vi "Main.vi"(11 "Module Admin":refnum<class "Delacor_lib_QMH_Module Admin.lvclass">) -> ()   [LabVIEW 2021, in "RT Interpreter.lvlib"]
doc: "This template is based off of the Queued Message Handler design pattern and the Queued Message Handler project template that ships with LabVIEW.\n\nThe main difference is that the queue is private to this module and communication between modules is performed via Broadcast and Request events.\n\nRequest events are wrapped in public API methods and are handled in the Event Handling Loop (EHL) of this VI. Any module can register for Broadcast events sent by this module. The EHL generates messages based on user interface actions.\n\nThe Message Handling Loop (MHL) processes messages generated by the EHL, or by other messages. The messages are string values, so new messages can be added easily to the Message Cases case structure in the MHL. Each message cluster can also provide an optional value for Message Data, which is a variant that can be converted to whatever message-specific data is required.\n_____\nBased on DQMH Dev Tools: Project Template 7.1.2.1547."
uses:
  RT Interpreter.lvlib
  <vilib>/Delacor/Delacor QMH/Libraries/Module Admin_class/Delacor_lib_QMH_Module Admin.lvclass
  Host/Host Interpreter/Host Initialization--cluster.ctl
  Module Data--cluster.ctl
  Stop Argument--cluster.ctl
  <vilib>/Delacor/Delacor QMH/Libraries/Message Queue_class/Delacor_lib_QMH_Message Queue.lvclass/Delacor_lib_QMH_Message Queue.ctl
  <vilib>/Delacor/Delacor QMH/Libraries/Module Admin_class/Delacor_lib_QMH_Module Admin.lvclass/Delacor_lib_QMH_Module Admin.ctl
  189c6fa9-2a90-4507-a0f2-9e31c6cf4c77.vi
  <vilib>/Delacor/Delacor QMH/Libraries/Message Queue_class/Delacor_lib_QMH_Enqueue Message (Single).vi
  <vilib>/Delacor/Delacor QMH/Libraries/Module Admin_class/Delacor_lib_QMH_Get External Launch.vi
  <vilib>/JDP Science/JSONtext/JSON text to Variant.vi
  <vilib>/JDP Science/JSONtext/LVClass Serializer/JSONtext LVClass Serializer.lvclass
  <vilib>/Delacor/Delacor QMH/Libraries/Message Queue_class/Delacor_lib_QMH_Message Queue.lvclass
  Libraries/UDP Comms/UDP Comms.lvlib
panel:
  out "Data out":T1
  out "error out":errorcluster
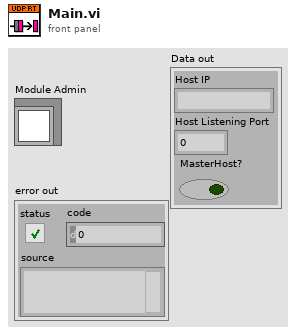
[diagram p1: front panel]
types:
  T1 = typedef "UDP Comms.lvlib/Host Initialization--cluster.ctl" = cluster{"Host IP":string, "Host Listening Port":u16, "MasterHost?":bool}
  T2 = typedef "RT Interpreter.lvlib/Request Events--cluster.ctl" = cluster{"Stop Module":refnum<user-event>, "Show Panel":refnum<user-event>, "Hide Panel":refnum<user-event>, "Get Module Execution Status":refnum<user-event>, "Show Diagram":refnum<user-event>, "Private.Open Connection":refnum<user-event>, "Private.Start Helper Loop":refnum<user-event>}
  T3 = typedef "RT Interpreter.lvlib/Module Data--cluster.ctl" = cluster{"IP Host":string, "Port RT":u16, "Port Host":u16, "connection ID":refnum<k16>}
  T4 = enum32{"invalid lock state", "Not Locked", "Locked (No Password)", "Password-protected"}
  T5 = typedef "RT Interpreter.lvlib/Stop Argument--cluster.ctl" = cluster{"Origin":string, "Exit via Stop Module Req?":bool, "Wait for Module to stop?":bool}
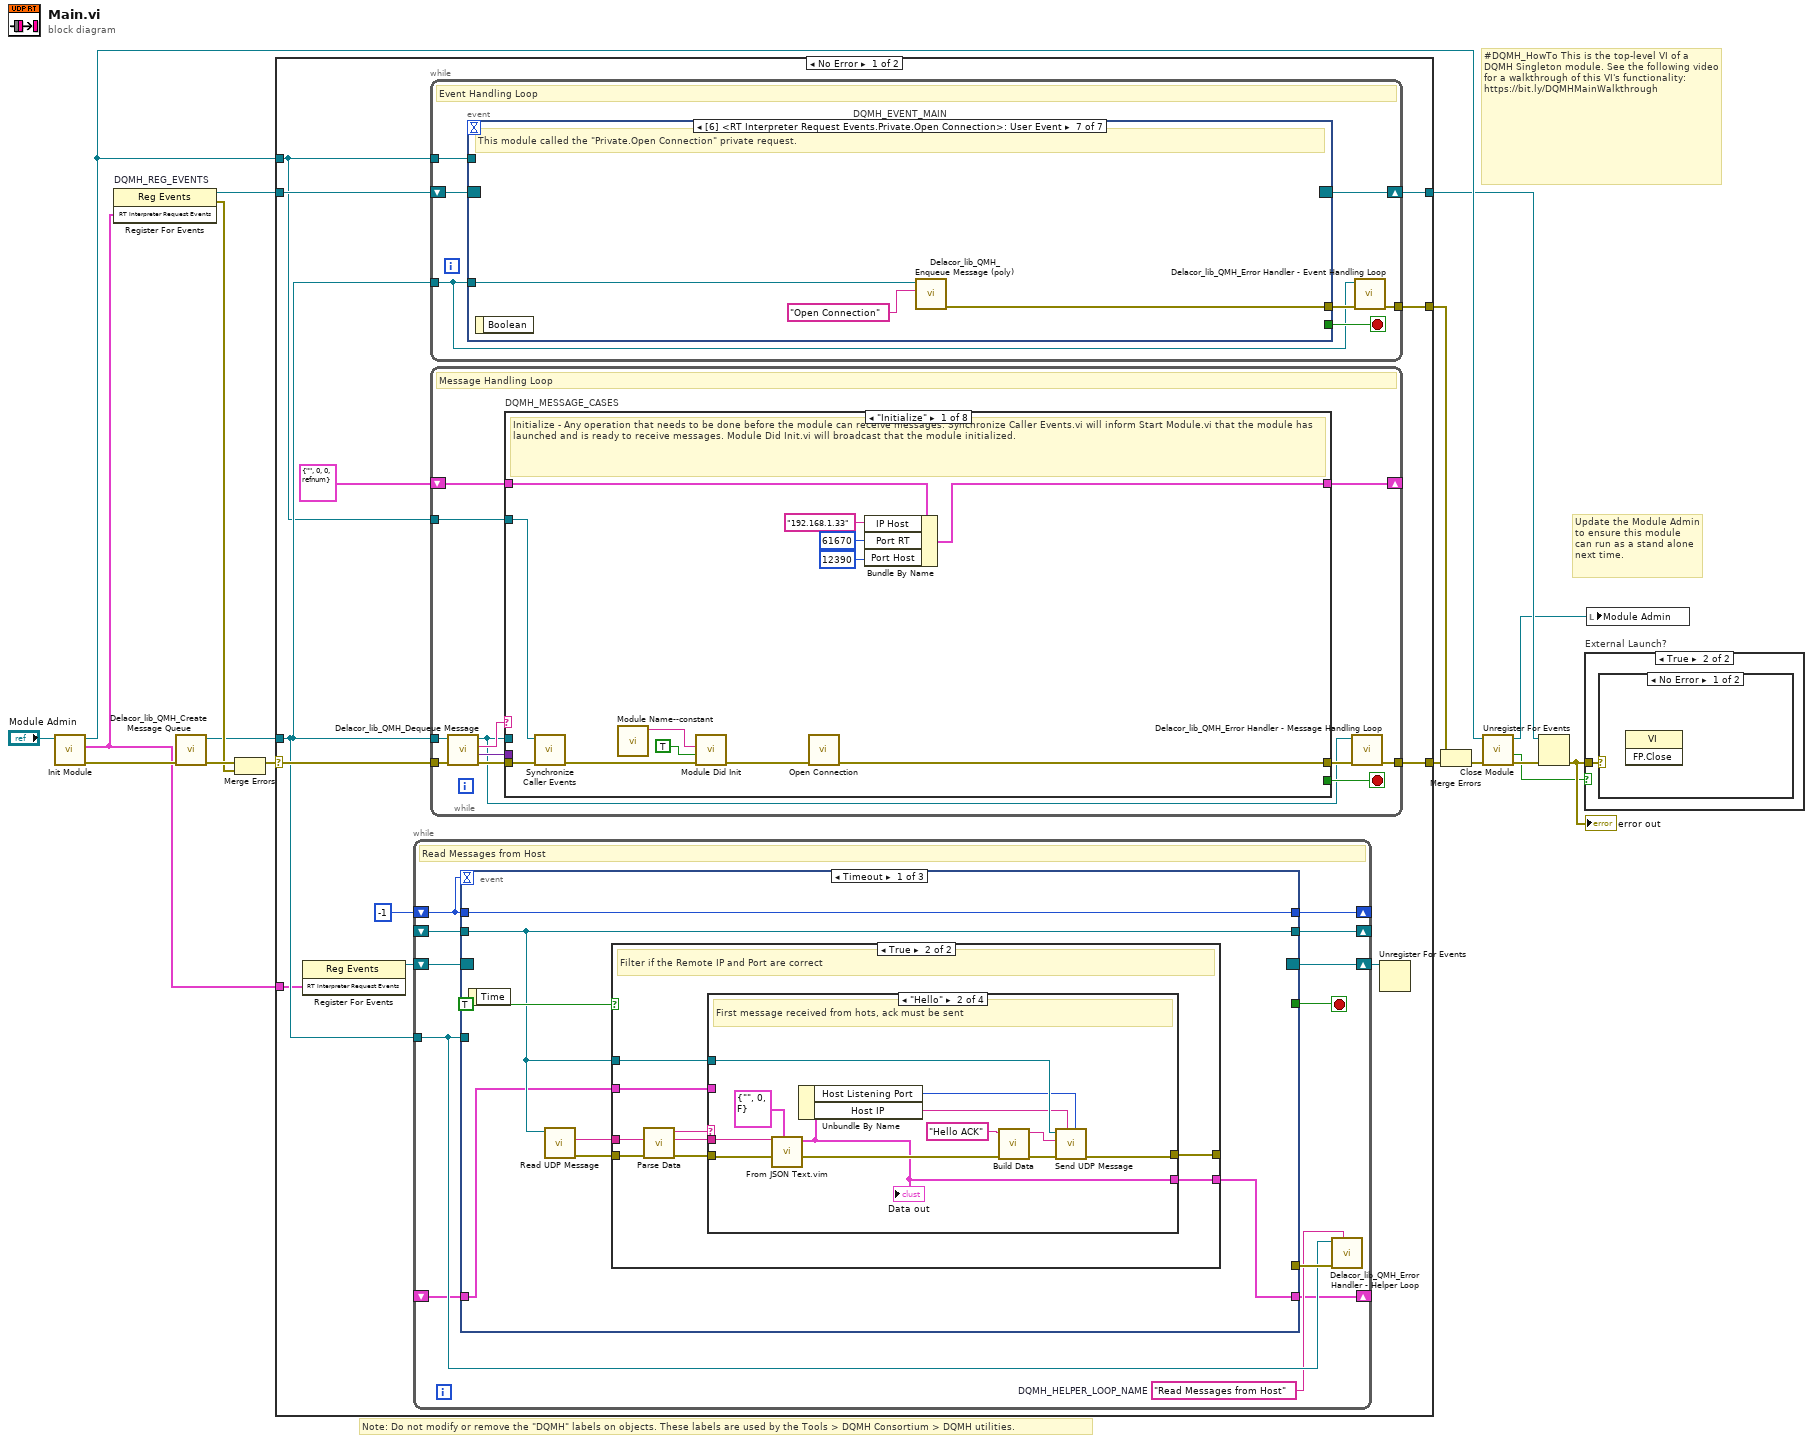
[diagram p0: block diagram]
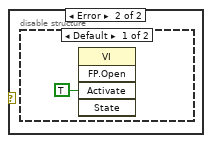
[diagram p3: hidden frame]
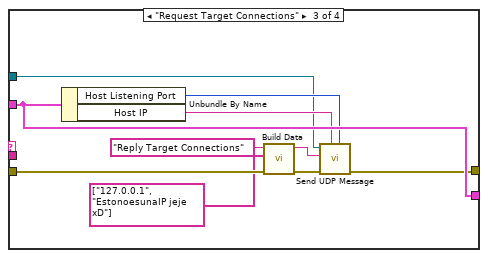
[diagram p7: hidden frame]
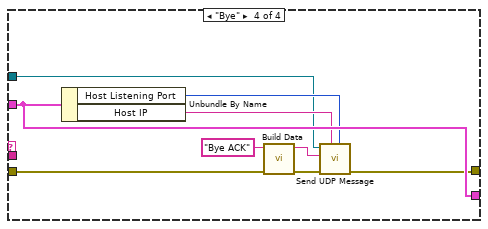
[diagram p8: hidden frame]
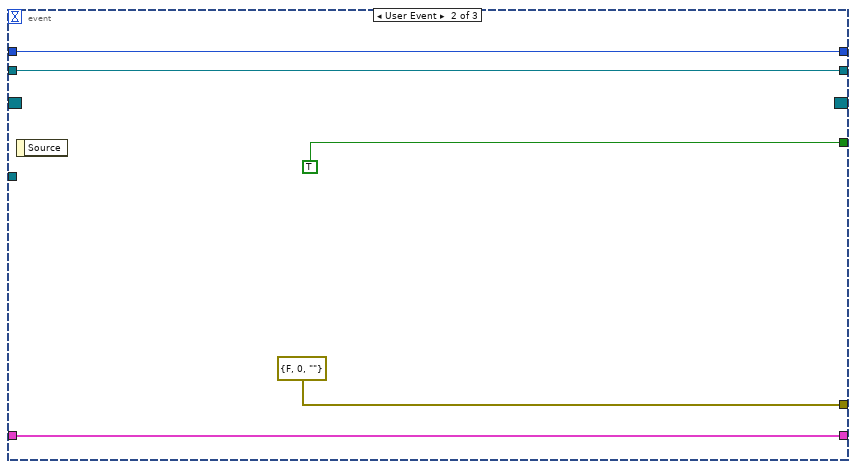
[diagram p9: hidden frame]
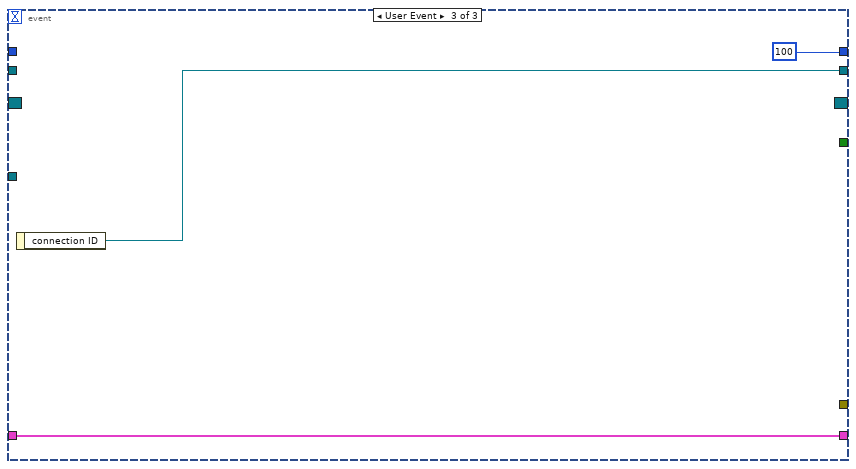
[diagram p10: hidden frame]
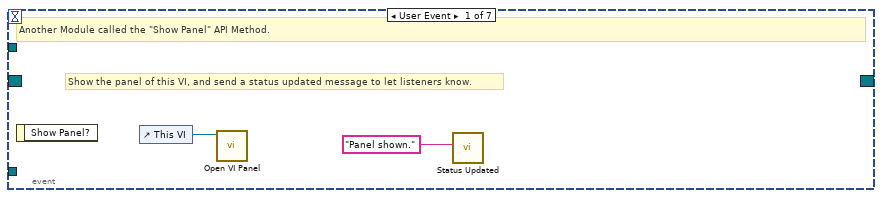
[diagram p11: hidden frame]
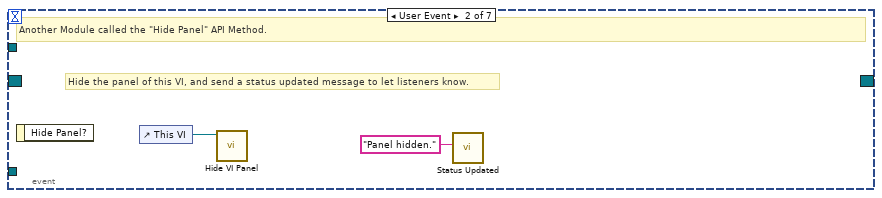
[diagram p12: hidden frame]
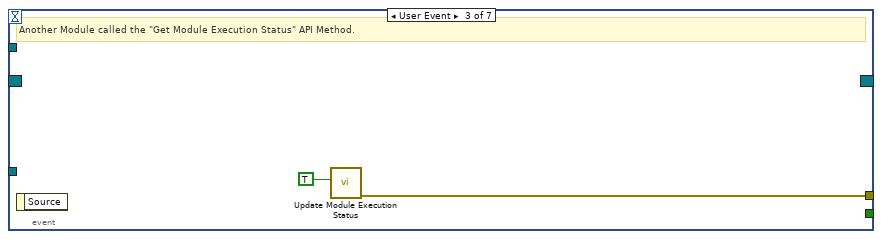
[diagram p13: hidden frame]
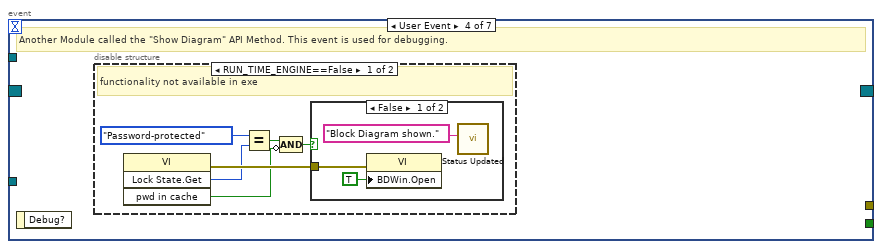
[diagram p14: hidden frame]
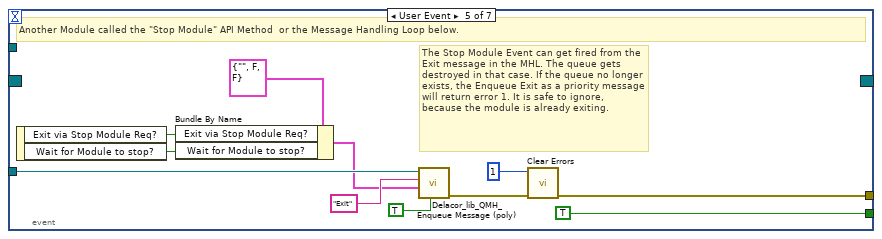
[diagram p17: hidden frame]
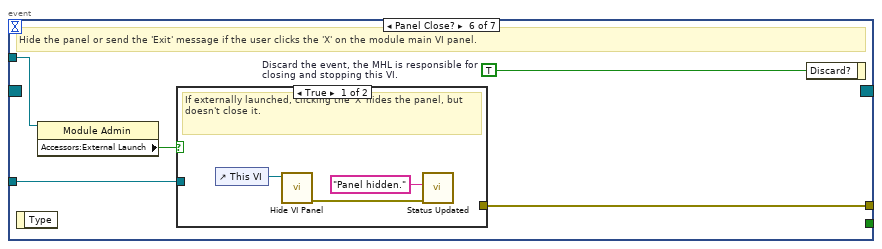
[diagram p18: hidden frame]
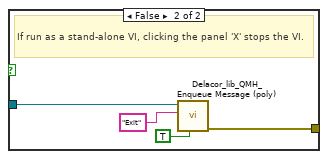
[diagram p19: hidden frame]
diagram:
  # "#DQMH_HowTo This is the top-level VI of a DQMH Singleton module. See the following video for a walkthrough of this VI's functionality: https://bit.ly/DQMHMainWalkthrough"
  # "Note: Do not modify or remove the \"DQMH\" labels on objects. These labels are used by the Tools > DQMH Consortium > DQMH utilities."
  # "Update the Module Admin to ensure this module can run as a stand alone next time."
  n1 = call "Init Module.vi"("Singleton Module Admin in"="Module Admin") -> ("error out"=w16:errorcluster, "RT Interpreter Request Events"=w1:T2, "Singleton Module Admin out"=w8:refnum<class "Delacor_lib_QMH_Module Admin.lvclass">)  [unwired: 8 in]
  n2 = register-events "DQMH_REG_EVENTS"(w1) -> (reference out=w6:refnum<event-registration>, error out=w9:errorcluster)  [unwired: 2 in]
  n3 = call <vilib>:"Delacor_lib_QMH_Create Message Queue.vi"("error in"=w16) -> ("error out"=w11:errorcluster, "Message Queue"=w5:refnum<class "Delacor_lib_QMH_Message Queue.lvclass">)  [unwired: 9 in]
  n4 = Merge Errors(w11, w9) -> (w10:errorcluster)
  n5 = case shown="No Error" w10 {
    selector: w10 -> [w27 w237]
    tunnel: [w29 w236] -> w17
    tunnel: [w26 w235] -> w7
    tunnel: w6 -> [w24 w235]
    tunnel: w5 -> [w23 w230]
    tunnel: [w28 _] -> w14
    tunnel: w8 -> [w22 w231]
    tunnel: w1 -> [w21 _]
    frame No Error {
      n6 = register-events ("DQMH_HELPER_REGFOREVENTS")(w21) -> (reference out=w19:refnum<event-registration>)  [unwired: 2 in, 1 out]
      n7 = while "DQMH_HELPER_LOOP" {
        shift-right: [w41] -> _
        shift-left: -1 -> [w40]
        shift-right: [w38] -> w20
        shift-left: w19 -> [w39]
        tunnel: w23 -> [w35]
        shift-right: [w33] -> _
        shift-left: _ -> [w32]
        shift-right: [w31] -> _
        shift-left: _ -> [w30]
        stop <- w37 stop-if-true
        w34 = "Read Messages from Host"  # DQMH_HELPER_LOOP_NAME
        # "Read Messages from Host"
        n8 = event "DQMH_HELPER_EVENT_STRUCTURE" shown="[0] Timeout" {
          selector: w39 -> [_ _ _]
          dyn-events: [_ _ _] -> w38
          timeout: w40 -> [_ _ _]
          tunnel: w40 -> [w48 w95 _]
          tunnel: [w48 w95 100] -> w41
          tunnel: [_ TRUE _] -> w37
          tunnel: [_ errorcluster {"status"=FALSE, "code"=0, "source"=""} ("error constant") _] -> w36
          tunnel: w35 -> [_ _ _]
          tunnel: [w44 w92 w98] -> w33
          tunnel: w32 -> [w44 w92 _]
          tunnel: [w43 w91 w96] -> w31
          tunnel: w30 -> [w42 w91 w96]
          event Timeout {
            n9 = event-data() -> ()  [unwired: 1 in, 1 out]
            n10 = call "Read UDP Message.vi"("Local UDP connection ref"=w44) -> ("error out"=w47:errorcluster, "data out"=w46:string)  [unwired: 7 in, 2 out]
            n11 = case shown="True" TRUE {
              tunnel: w47 -> [_ w58]
              tunnel: w46 -> [_ w57]
              tunnel: [_ w53] -> _
              tunnel: w44 -> [_ w52]
              tunnel: [w49 w51] -> w43
              tunnel: w42 -> [w49 w50]
              frame False {
              }
              frame True {
                # "Filter if the Remote IP and Port are correct"
                n12 = call "Parse Data.vi"("error in (no error)"=w58, "Received UDP Data"=w57) -> ("error out"=w55:errorcluster, "Data"=w54:string, "Command"=w56:string)  [unwired: 7 in]
                n13 = case shown="\"Hello\"" w56 {
                  tunnel: w55 -> [_ w70 w80 w89]
                  tunnel: w54 -> [_ w69 _ _]
                  tunnel: [_ w61 w78 w87] -> w53
                  tunnel: w52 -> [_ w64 w72 w82]
                  tunnel: [w59 w60 w81 w90] -> w51
                  tunnel: w50 -> [w59 _ w81 w90]
                  frame Default {
                  }
                  frame "Hello" {
                    # "First message received from hots, ack must be sent"
                    n14 = call "From JSON Text.vim"("Data Type and Default Value"=T1 {"Host IP"="", "Host Listening Port"=0, "MasterHost?"=FALSE} ("Host Initialization--cluster"), "error in (no error)"=w70, "JSON"=w69) -> ("error out"=w67:errorcluster, "Data out"=w60:T1)  [unwired: 7 in]
                    "Data out" <- w60
                    n15 = Unbundle By Name(w60) -> ("Host Listening Port"=w62:u16, "Host IP"=w63:string)
                    n16 = call "Build Data.vi"("error in (no error)"=w67, "Command"="Hello ACK") -> ("error out"=w65:errorcluster, "UDP MSG To be Sent"=w66:string)  [unwired: 8 in]
                    n17 = call "Send UDP Message.vi"("Remote UDP Listening Port"=w62, "Remote IP"=w63, "error in"=w65, "UDP Data to be sent"=w66, "Local UDP connection ref"=w64) -> ("error out"=w61:errorcluster)  [unwired: 5 in, 1 out]
                  }
                  frame "Request Target Connections" {
                    n18 = Unbundle By Name(w81) -> ("Host Listening Port"=w76:u16, "Host IP"=w77:string)
                    n19 = call "Build Data.vi"("error in (no error)"=w80, "Data"=string[] ["127.0.0.1", "EstonoesunaIP jeje xD"], "Command"="Reply Target Connections") -> ("error out"=w79:errorcluster, "UDP MSG To be Sent"=w73:string)  [unwired: 7 in]
                    n20 = call "Send UDP Message.vi"("Remote UDP Listening Port"=w76, "Remote IP"=w77, "error in"=w79, "UDP Data to be sent"=w73, "Local UDP connection ref"=w72) -> ("error out"=w78:errorcluster)  [unwired: 5 in, 1 out]
                  }
                  frame "Bye" {
                    n21 = Unbundle By Name(w90) -> ("Host Listening Port"=w85:u16, "Host IP"=w86:string)
                    n22 = call "Build Data.vi"("error in (no error)"=w89, "Command"="Bye ACK") -> ("error out"=w88:errorcluster, "UDP MSG To be Sent"=w83:string)  [unwired: 8 in]
                    n23 = call "Send UDP Message.vi"("Remote UDP Listening Port"=w85, "Remote IP"=w86, "error in"=w88, "UDP Data to be sent"=w83, "Local UDP connection ref"=w82) -> ("error out"=w87:errorcluster)  [unwired: 5 in, 1 out]
                  }
                }
              }
            }
          }
          event User Event {
            n24 = event-data() -> ()  [unwired: 1 in, 1 out]
          }
          event User Event {
            n25 = event-data() -> ("connection ID"=w98:refnum<k16>)  [unwired: 1 in]
          }
        }
        n26 = call-dynamic "Delacor_lib_QMH_Error Handler - Helper Loop.vi"("Error Debug"=w34, "error in"=w36, "Message Queue in"=w35) -> ()  [unwired: 7 in, 2 out]
      }
      n27 = while {
        tunnel: w23 -> [w99]
        shift-right: [w102] -> w26
        shift-left: w24 -> [w103]
        tunnel: [w104] -> w28
        tunnel: w22 -> [w100]
        stop <- w101 stop-if-true
        # "Event Handling Loop"
        n28 = event "DQMH_EVENT_MAIN" shown="[6] <RT Interpreter Request Events.Private.Open Connection>: User Event" {
          selector: w103 -> [_ _ _ _ _ _ _]
          dyn-events: [_ _ _ _ _ _ _] -> w102
          timeout: _ -> [_ _ _ _ _ _ _]
          tunnel: [_ _ _ _ TRUE ("Discard?") _ _] -> w101
          tunnel: w99 -> [_ _ _ _ w127 w134 w146]
          tunnel: [_ _ w111 _ w130 w136 w144] -> w105
          tunnel: w100 -> [_ _ _ _ _ w133 _]
          event User Event {
            # "Show the panel of this VI, and send a status updated message to let listeners know."
            # "Another Module called the \"Show Panel\" API Method."
            n29 = event-data() -> ()  [unwired: 1 in, 1 out]
            n30 = control-ref of="This VI"() -> (w107:refnum<vi>)
            n31 = call "Open VI Panel.vi"("VI"=w107) -> ()  [unwired: 10 in, 1 out]
            n32 = call "Status Updated.vi"("Status"="Panel shown." ("format string")) -> ()  [unwired: 10 in, 1 out]
          }
          event User Event {
            # "Hide the panel of this VI, and send a status updated message to let listeners know."
            # "Another Module called the \"Hide Panel\" API Method."
            n33 = event-data() -> ()  [unwired: 1 in, 1 out]
            n34 = control-ref of="This VI"() -> (w109:refnum<vi>)
            n35 = call "Hide VI Panel.vi"("VI"=w109) -> ()  [unwired: 10 in, 1 out]
            n36 = call "Status Updated.vi"("Status"="Panel hidden." ("format string")) -> ()  [unwired: 10 in, 1 out]
          }
          event User Event {
            # "Another Module called the \"Get Module Execution Status\" API Method."
            n37 = event-data() -> ()  [unwired: 1 in, 1 out]
            n38 = call "Update Module Execution Status.vi"("Running?"=TRUE) -> ("error out"=w111:errorcluster)  [unwired: 10 in]
          }
          event User Event {
            # "Another Module called the \"Show Diagram\" API Method. This event is used for debugging."
            n39 = event-data() -> ()  [unwired: 1 in, 1 out]
            n40 = disable-structure shown="RUN_TIME_ENGINE==False" {
              frame condition #0 (active) {
                # "functionality not available in exe"
                n41 = invoke on="Invoke Node" class="VI" method="Lock State.Get"() -> (error out=w117:errorcluster, "Get Lock State"=w116:T4, "pwd in cache"=w113:bool)  [unwired: 4 in, 1 out]
                n42 = Equal?(x=T4."Password-protected", y=w116) -> (x = y?=w114:bool)
                n43 = Compound Arithmetic op=AND(w114, invert w113) -> (w112:bool)
                n44 = case shown="False" w112 {
                  tunnel: w117 -> [w120 _]
                  frame False {
                    n45 = property on="Property Node" class="VI"(error in=w120, "BDWin.Open"=TRUE ("Block Diagram Window:Open")) -> ()  [unwired: 1 in, 2 out]
                    n46 = call "Status Updated.vi"("Status"="Block Diagram shown." ("format string")) -> ()  [unwired: 10 in, 1 out]
                  }
                  frame True {
                    # "Password-protected VI, and the password is not in the cache. Do not show the diagram."
                  }
                }
              }
              frame condition #1 {
              }
            }
          }
          event User Event {
            # "The Stop Module Event can get fired from the Exit message in the MHL. The queue gets destroyed in that case. If the queue no longer exists, the Enqueue Exit as a priority message will return error 1. It is safe to ignore, because the module is already exiting."
            # "Another Module called the \"Stop Module\" API Method  or the Message Handling Loop below."
            n47 = event-data() -> ("Exit via Stop Module Req?"=w123:bool, "Wait for Module to stop?"=w122:bool)  [unwired: 1 in]
            n48 = Bundle By Name(cluster=T5 {"Origin"="", "Exit via Stop Module Req?"=FALSE, "Wait for Module to stop?"=FALSE} ("Stop Argument"), "Exit via Stop Module Req?"=w123, "Wait for Module to stop?"=w122) -> (w121:T5)
            n49 = call-poly <vilib>:"Delacor_lib_QMH_Enqueue Message (poly).vi"("Priority Message? (F)"=TRUE, "Message Data"=w121, "Message"="Exit", "Message Queue in"=w127) -> ("error out"=w131:errorcluster)  [unwired: 6 in, 1 out]
            n50 = call <vilib>:"Clear Errors.vi"("error in (no error)"=w131, "specific error code to clear (0: all)"=1) -> ("error out"=w130:errorcluster)  [unwired: 4 in, 1 out]
          }
          event Panel Close? {
            w135 = TRUE  # Discard the event, the MHL is responsible for closing and stopping this VI.
            # "Hide the panel or send the 'Exit' message if the user clicks the 'X' on the module main VI panel."
            n51 = event-data() -> ()  [unwired: 1 in, 1 out]
            n52 = property on="Property Node" class="Module Admin"(reference=w133) -> ("Accessors:External Launch"=w132:bool)  [unwired: 1 in, 2 out]
            n53 = case shown="True" w132 {
              tunnel: w134 -> [_ w142]
              tunnel: [_ w143] -> w136
              frame True {
                # "If externally launched, clicking the 'X' hides the panel, but doesn't close it."
                n54 = control-ref of="This VI"() -> (w139:refnum<vi>)
                n55 = call "Hide VI Panel.vi"("VI"=w139) -> ("error out"=w137:errorcluster)  [unwired: 10 in]
                n56 = call "Status Updated.vi"("error in"=w137, "Status"="Panel hidden." ("format string")) -> ()  [unwired: 9 in, 1 out]
              }
              frame False {
                # "If run as a stand-alone VI, clicking the panel 'X' stops the VI."
                n57 = call-poly <vilib>:"Delacor_lib_QMH_Enqueue Message (poly).vi"("Priority Message? (F)"=TRUE, "Message"="Exit", "Message Queue in"=w142) -> ("error out"=w143:errorcluster)  [unwired: 7 in, 1 out]
              }
            }
            n58 = event-data ("Event Filter Node")("Discard?"=w135) -> ()  [unwired: 1 in, 1 out]
          }
          event User Event {
            # "This module called the \"Private.Open Connection\" private request."
            n59 = event-data() -> ()  [unwired: 1 in, 1 out]
            n60 = call-poly <vilib>:"Delacor_lib_QMH_Enqueue Message (poly).vi"("Message"="Open Connection", "Message Queue in"=w146) -> ("error out"=w144:errorcluster)  [unwired: 8 in, 1 out]
          }
        }
        n61 = call-dynamic "Delacor_lib_QMH_Error Handler - Event Handling Loop.vi"("error in"=w105, "Message Queue in"=w99) -> ("dup error in"=w104:errorcluster)  [unwired: 8 in, 1 out]
      }
      n62 = while {
        tunnel: w23 -> [w147]
        shift-right: [w155] -> _
        shift-left: T3 {"IP Host"="", "Port RT"=0, "Port Host"=0, "connection ID"=refnum} ("Data Cluster") -> [w156]
        tunnel: w27 -> [w158]
        tunnel: [w150] -> w29
        tunnel: w22 -> [w151]
        stop <- w154 stop-if-true
        # "Message Handling Loop"
        n63 = call-dynamic "Delacor_lib_QMH_Dequeue Message.vi"("error in"=w158, "Message Queue in"=w147) -> ("error out"=w157:errorcluster, "Message Data"=w152:variant, "Message"=w153:string, "Message Queue out"=w148:refnum<class "Delacor_lib_QMH_Message Queue.lvclass">)  [unwired: 6 in]
        n64 = case "DQMH_MESSAGE_CASES" shown="\"Initialize\"" w153 {
          selector: w153 -> [_ _ _ _ _ _ _ w225]
          tunnel: w148 -> [_ _ _ _ _ w190 w213 _]
          tunnel: w157 -> [w170 w172 w181 w184 w186 w197 w219 w228]
          tunnel: [w164 w172 w175 w183 w186 w193 w214 w229] -> w149
          tunnel: w156 -> [w162 w171 w178 w182 w185 w192 w205 w226]
          tunnel: [w163 w171 w174 w182 w185 w192 w205 w226] -> w155
          tunnel: [_ _ _ _ _ _ w212 _] -> w154
          tunnel: w152 -> [_ _ _ _ _ w191 w211 _]
          tunnel: w151 -> [w168 _ _ _ _ w189 w206 _]
          frame "Initialize" {
            # "Initialize - Any operation that needs to be done before the module can receive messages. Synchronize Caller Events.vi will inform Start Module.vi that the module has launched and is ready to receive messages. Module Did Init.vi will broadcast that the module initialized."
            n65 = call "Synchronize Caller Events.vi"("error in"=w170, "Singleton Module Admin in"=w168) -> ("error out"=w169:errorcluster)  [unwired: 8 in, 1 out]
            n66 = call "Module Name--constant.vi"() -> ("Module Name"=w166:string)  [unwired: 11 in]
            n67 = call "Module Did Init.vi"("error in"=w169, "Initialized?"=TRUE, "Origin"=w166) -> ("error out"=w165:errorcluster)  [unwired: 8 in]
            n68 = call "Open Connection.vi"("error in"=w165) -> ("error out"=w164:errorcluster)  [unwired: 10 in]
            n69 = Bundle By Name(cluster=w162, "IP Host"="192.168.1.33", "Port RT"=u16 61670, "Port Host"=u16 12390) -> (w163:T3)
          }
          frame "---Module Specific---" {
            # "Separator -- The following cases handle messages specific to this Module."
          }
          frame "Open Connection" {
            n70 = Unbundle By Name(w178) -> ("Port RT"=w177:u16)
            n71 = UDP Open(8:w181, 11:w177) -> (port=w173:refnum<k16>, 0:w180:errorcluster)  [unwired: 3 in, 1 out]
            n72 = Bundle By Name(cluster=w178, "connection ID"=w173) -> (w174:T3)
            n73 = call "Start Helper Loop.vi"("connection ID"=w173) -> ()  [unwired: 10 in, 1 out]
            n74 = call "Status Updated.vi"("error in"=w180, "Status"="Open UDP Connection Successfully") -> ("error out"=w176:errorcluster)  [unwired: 9 in]
            n75 = call "Send UDP Info to TL.vi"("error in"=w176, "UDP Info"=w174) -> ("error out"=w175:errorcluster)  [unwired: 9 in]
          }
          frame "---Copy This Frame---" {
            # "Duplicate this frame when creating new messages.  Change this comment in the duplicated frame to describe this message."
            n76 = Merge Errors(w184) -> (w183:errorcluster)
          }
          frame "---Exit and Error Handling---" {
            # "Separator - The following cases handle errors and exit messages."
          }
          frame "Error" {
            # "#DQMH_CodeRecommended - If the module is running in standalone mode (External Launch = FALSE), this code will pop up an error dialog and call the 'Exit' message if an error occurs. Add more fine-grained error management here."
            # "Error - Check the error message data and respond accordingly. This message is sent by the \"Error Handler\" VIs at the end of each loop in this application."
            n77 = property on="Property Node" class="Module Admin"(reference=w189) -> ("Accessors:External Launch"=w188:bool)  [unwired: 1 in, 2 out]
            n78 = Variant To Data(error in=w197, type=errorcluster {"status"=FALSE, "code"=0, "source"=""} ("error constant"), Variant=w191) -> (data=w187:errorcluster, error out=w195:errorcluster)
            n79 = local write "error out"(w187) -> ()
            n80 = call "Error Reported.vi"("Error"=w187) -> ()  [unwired: 10 in, 1 out]
            n81 = case shown="False" w188 {
              tunnel: [w202 _] -> w194
              tunnel: w190 -> [w200 _]
              tunnel: w187 -> [w201 _]
              frame False {
                n82 = disable-structure shown="Default" {
                  disable-tunnel: w201 -> [w203 _]
                  frame condition #0 (active) {
                    # "If the module is running standalone, then pop up an error dialog and call the \"Exit\" message."
                    n83 = call <vilib>:"Simple Error Handler.vi"("error in (no error)"=w203) -> ()  [unwired: 4 in, 5 out]
                  }
                  frame condition #1 {
                    # "To prevent the Simple Error Handler VI from being loaded (e.g. when deploying to a Real-Time target), add the Conditional Disable Symbol \"DQMH_Disable_SEH\" to your project and set it to TRUE."
                  }
                }
                n84 = call-poly <vilib>:"Delacor_lib_QMH_Enqueue Message (poly).vi"("Priority Message? (F)"=TRUE, "Message"="Exit", "Message Queue in"=w200) -> ("error out"=w202:errorcluster)  [unwired: 7 in, 1 out]
              }
              frame True {
                # "If the module was launched externally, calling the Error Reported broadcast VI is the only action performed by the \"Error\" message. The module's caller can then process the error appropriately."
              }
            }
            n85 = Merge Errors(w195, w194) -> (w193:errorcluster)
          }
          frame "Exit" {
            w210 = 91  # 91: not all Exit messages will have an argument
            w212 = TRUE  # Stop the VI
            # "Release the message queue reference"
            # "Exit - Exit the application."
            n86 = Variant To Data(error in=w219, type=T5 {"Origin"="", "Exit via Stop Module Req?"=FALSE, "Wait for Module to stop?"=FALSE} ("Stop Argument"), Variant=w211) -> (data=w208:T5, error out=w216:errorcluster)
            n87 = call <vilib>:"Clear Errors.vi"("error in (no error)"=w216, "specific error code to clear (0: all)"=w210) -> ("error out"=w218:errorcluster)  [unwired: 4 in, 1 out]
            n88 = control-ref of="This VI"() -> (w207:refnum<vi>)
            n89 = call-dynamic "Delacor_lib_QMH_Release Message Queue.vi"("error in"=w218, "Message Queue"=w213) -> ("error out"=w217:errorcluster)  [unwired: 9 in]
            n90 = call "Handle Exit.vi"("Stop Argument"=w208, "Admin in"=w206, "VI reference"=w207) -> ("error out"=w215:errorcluster)  [unwired: 7 in, 1 out]
            n91 = Merge Errors(w217, w215) -> (w214:errorcluster)
            n92 = Unbundle By Name(w205) -> ("connection ID"=w204:refnum<k16>)
            n93 = call "Error Reported.vi"("Error"=w214) -> ()  [unwired: 10 in, 1 out]
            n94 = UDP Close(connection ID=w204) -> ()  [unwired: 1 in, 2 out]
          }
          frame Default {
            # "'Default' case only runs if there is a message that isn't defined in any of the other cases.  Output a programming error."
            n95 = call "Module Name--constant.vi"() -> ("Module Name"=w224:string)  [unwired: 11 in]
            n96 = Format Into String(format string="The invalid message string \"%s\" was received in the Message Handling Loop for module \"%s\".", w225, w224) -> (resulting string=w220:string)  [unwired: 2 in, 1 out]
            n97 = call <vilib>:"Error Cluster From Error Code.vi"("show call chain? (False)"=TRUE, "error message (\"\")"=w220, "error code (0)"=1) -> ("error out"=w227:errorcluster)  [unwired: 6 in]
            n98 = Merge Errors(w228, w227) -> (w229:errorcluster)
          }
        }
        n99 = call-dynamic "Delacor_lib_QMH_Error Handler - Message Handling Loop.vi"("error in"=w149, "Message Queue in"=w148) -> ("dup error in"=w150:errorcluster)  [unwired: 8 in, 1 out]
      }
      n100 = Unregister For Events(event registration refnum=w20) -> ()  [unwired: 1 in, 1 out]
    }
    frame Error {
      # "Synchronize Caller Events.vi will inform Start Module.vi that the module has launched and will let the code calling Start Module.vi register for broadcasts and would permit the caller receive the broadcast that an error occurred at launch time."
      n101 = call-dynamic "Delacor_lib_QMH_Release Message Queue.vi"("error in"=w237, "Message Queue"=w230) -> ("error out"=w236:errorcluster)  [unwired: 9 in]
      n102 = call "Synchronize Caller Events.vi"("Singleton Module Admin in"=w231) -> ("error out"=w238:errorcluster)  [unwired: 9 in, 1 out]
      n103 = call "Module Name--constant.vi"() -> ("Module Name"=w234:string)  [unwired: 11 in]
      n104 = Format Into String(format string="An error occurred during initialization. %s is no longer running.", w234) -> (resulting string=w232:string)  [unwired: 2 in, 1 out]
      n105 = Merge Errors(w236, w238) -> (w239:errorcluster)
      n106 = call "Error Reported.vi"("Additional Information"=w232, "Error"=w239) -> ()  [unwired: 9 in, 1 out]
    }
  }
  n107 = Merge Errors(w14, w17) -> (w13:errorcluster)
  n108 = call "Close Module.vi"("error in"=w13, "Module Admin in"=w8) -> ("error out"=w15:errorcluster, "External Launch"=w2:bool, "Module Admin out"=w3:refnum<class "Delacor_lib_QMH_Module Admin.lvclass">)  [unwired: 7 in]
  n109 = Unregister For Events(event registration refnum=w7, error in=w15) -> (error out=w12:errorcluster)
  "error out" <- w12
  n110 = case "External Launch?" shown="True" w2 {
    tunnel: w12 -> [_ w240]
    frame False {
    }
    frame True {
      n111 = case shown="No Error" w240 {
        frame No Error {
          n112 = invoke on="Invoke Node" class="VI" method="FP.Close"() -> ()  [unwired: 3 in, 3 out]
        }
        frame Error {
          n113 = disable-structure shown="Default" {
            frame condition #0 (active) {
              n114 = invoke class="VI" method="FP.Open"("Activate"=TRUE ("Activate?")) -> ()  [unwired: 4 in, 5 out]
            }
            frame condition #1 {
              # "Don't show panel on error if running inside a built EXE."
            }
          }
        }
      }
    }
  }
  n115 = local write "Module Admin"(w3) -> ()
